vi "Polarplot.vi"(8 "maximum":dbl=300.0 format="%0.2f", 9 "dimensions (w,h)":cluster{"width":i16, "height":i16}, 10 "Direction":dbl[](array[numeric])=[0.0, 45.0, 90.0, 135.0, 180.0, 225.0, 270.0, 315.0, 360.0], 11 "Magnitude":dbl[](array[numeric])=[100.0, 200.0, 100.0, 300.0, 100.0, 300.0, 100.0, 200.0, 100.0]) -> (3 "Data Aquired":picture)   [LabVIEW 2012]
panel:
  in  "polar attributes":T1={"maximum"=300.0, "minimum"=0.0, "clip to min"=FALSE, "log?(F)"=FALSE, "grid color"=16777228, "plot color"=16711680, "fmt and prec"={"format"=enum."Decimal", "precision"=0}, "visible section"=8} {"minimum" format="%0.2f"; "maximum" format="%0.2f"}
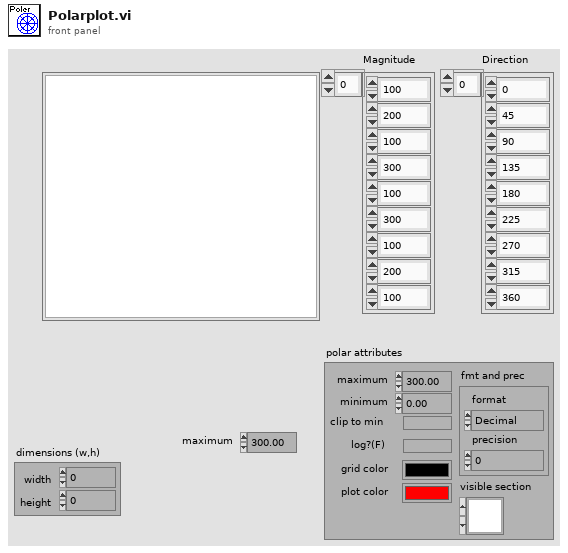
[diagram p1: front panel]
types:
  T1 = cluster{"maximum":dbl, "minimum":dbl, "clip to min":bool, "log?(F)":bool, "grid color":u32, "plot color":u32, "fmt and prec":cluster{"format":enum8{"Decimal", "Scientific", "Engineering", "Binary", "Octal", "Hex"}, "precision":u8}, "visible section":u16}
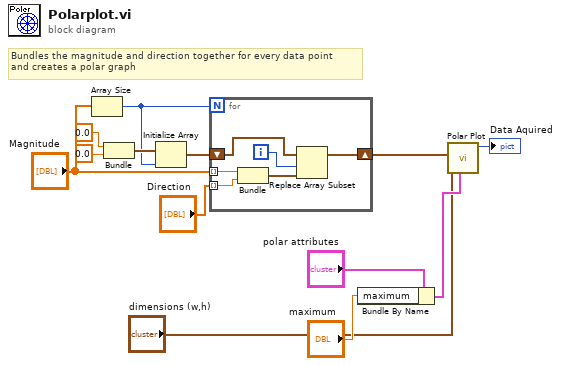
[diagram p0: block diagram]
diagram:
  # "Bundles the magnitude and direction together for every data point\nand creates a polar graph"
  n1 = Array Size(array="Magnitude") -> (size(s)=w7:i32)
  n2 = Bundle(0.0, 0.0) -> (w9:cluster{dbl, dbl})  [unwired: 1 in]
  n3 = Initialize Array(w9, w7) -> (w8:cluster{dbl, dbl}[])
  n4 = for {
    N: w7 -> [_]
    shift-right: [w15] -> w6
    shift-left: w8 -> [w16]
    tunnel: "Magnitude" -> [w19] mode=indexing
    tunnel: "Direction" -> [w18] mode=indexing
    i -> [w17]
    n5 = Bundle(w19, w18) -> (w14:cluster{dbl, dbl})  [unwired: 1 in]
    n6 = Replace Array Subset(array=w16, new element=w14, index=w17) -> (w15:cluster{dbl, dbl}[])
  }
  n7 = Bundle By Name(cluster="polar attributes", "maximum"="maximum") -> (w4:T1)
  n8 = call <vilib>:"Polar Plot.vi"("polar attributes"=w4, "dimensions (w,h)"="dimensions (w,h)", "data array [mag, phase (deg)]"=w6) -> ("new picture"=→"Data Aquired":picture)  [unwired: 8 in]
